vi "14.1 Floss Detection.vi"(8 "ErrI":errorcluster) -> (0 "ErrO":errorcluster)   [LabVIEW 2016]
uses:
  <vilib>/vision/Image Controls.llb/IMAQ Image.ctl
  <vilib>/vision/NI_Vision_Development_Module.lvlib
panel:
  out "Standard  Deviation":sgl format="%#_4g"
  out "Mean Intensity":sgl format="%#_4g"
  in  "Lower Deviation":sgl=64.0
  in  "Upper Deviation":sgl=68.0
  in  "Lower Mean Limitl":sgl=25.0
  in  "Upper Mean Intensity":sgl=28.0
  out "Image":T1(plugin-control)
  in  "Next":bool
  in  "Exit":bool
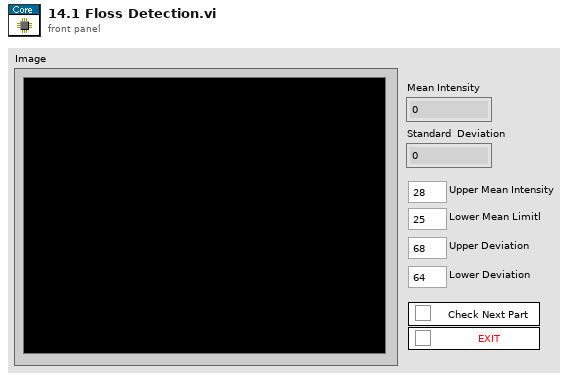
[diagram p1: front panel]
types:
  T1 = typedef "IMAQ Image.ctl" = refnum<image>
  T2 = typedef "IMAQ Rectangle" = cluster{"Left":i32, "Top":i32, "Right":i32, "Bottom":i32, "Rotation":dbl}
  T3 = typedef "IMAQ Coordinate System" = cluster{"Reference System":cluster{"Origin":cluster{"X":sgl, "Y":sgl}, "Angle (deg)":sgl, "Axis Reference":u32}, "Measurement System":cluster{"Origin":cluster{"X":sgl, "Y":sgl}, "Angle (deg)":sgl, "Axis Reference":u32}}
  T4 = cluster{"Tmp":T1, "Src":T1, "Parts":string[], "RefCoord":T3, "MsrCoord":T3, "MsrROI":T2}
  T5 = cluster{"Algorithm":i32, "Minimum Match Score":sgl, "SubPixel Accuracy":bool, "Rotation Angle Ranges":cluster{"Start":sgl, "End":sgl}[], "Show Search Area":bool, "Show Feature Found":bool, "Show Result":bool}
  T6 = cluster{"Mean Intensity":sgl, "Standard  Deviation":sgl, "Minimum Intensity":sgl, "Maximum Intensity":sgl}
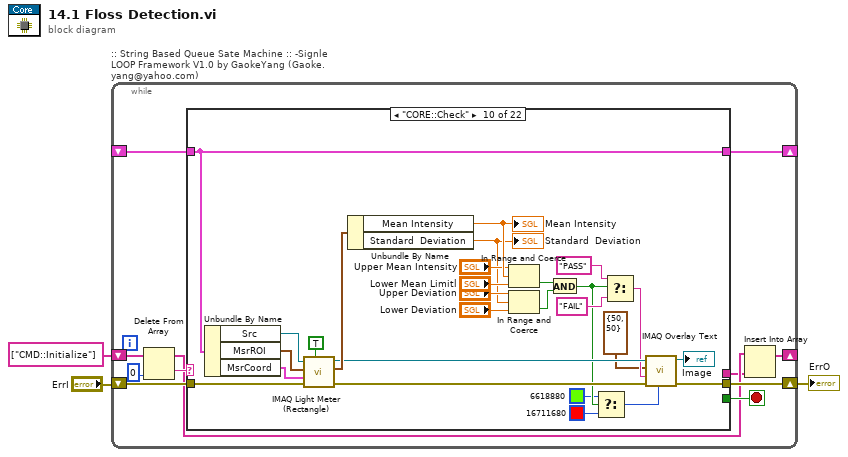
[diagram p0: block diagram]
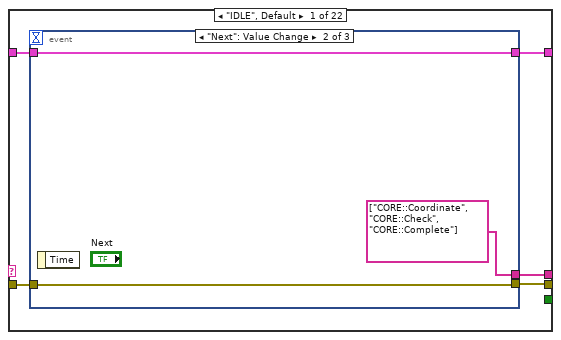
[diagram p2: hidden frame]
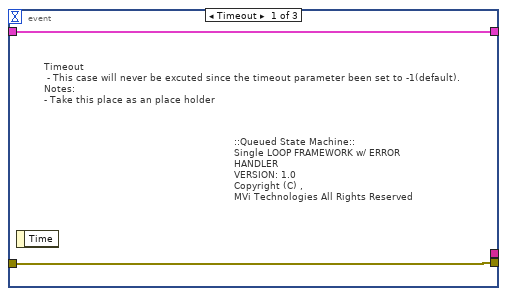
[diagram p3: hidden frame]
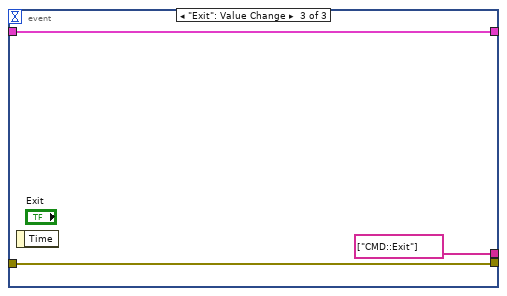
[diagram p4: hidden frame]
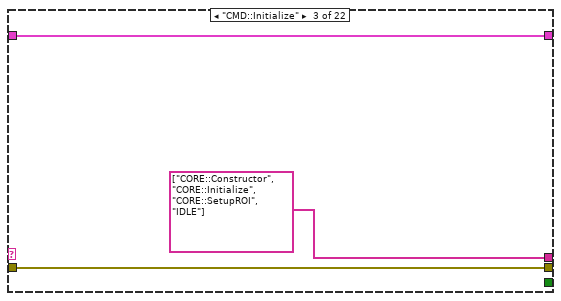
[diagram p6: hidden frame]
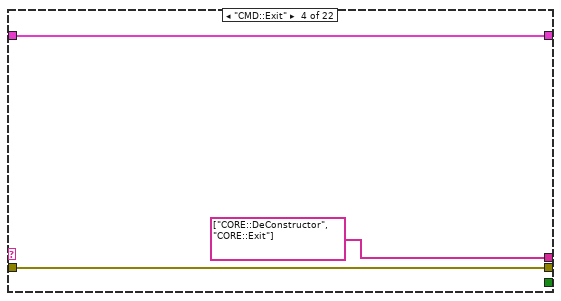
[diagram p7: hidden frame]
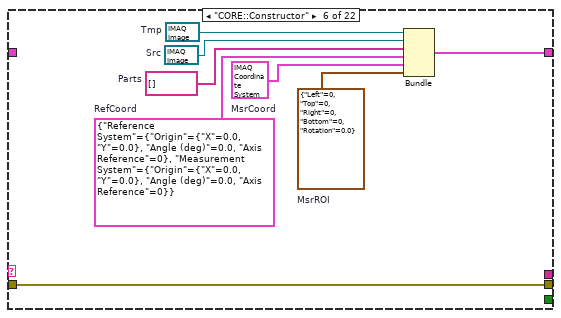
[diagram p9: hidden frame]
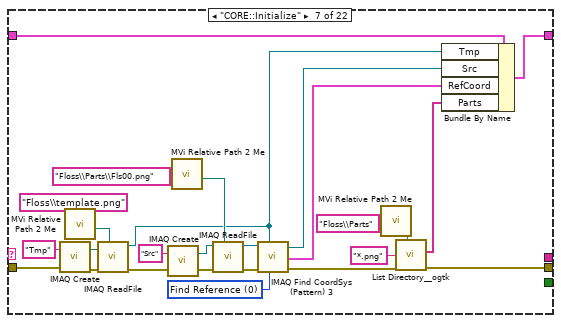
[diagram p10: hidden frame]
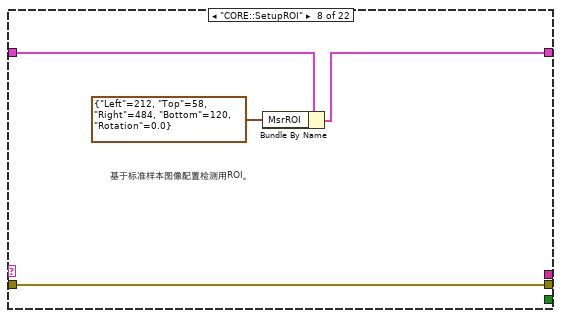
[diagram p11: hidden frame]
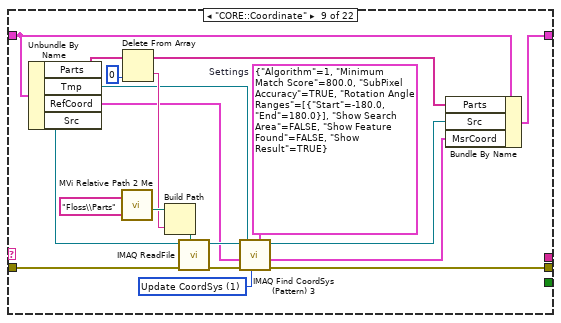
[diagram p12: hidden frame]
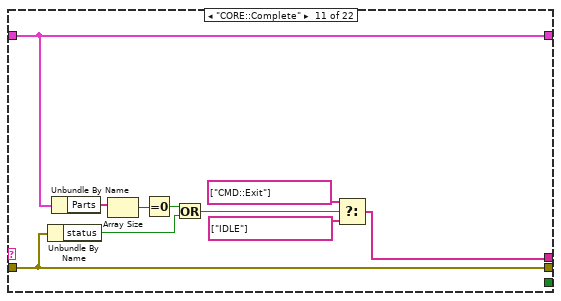
[diagram p13: hidden frame]
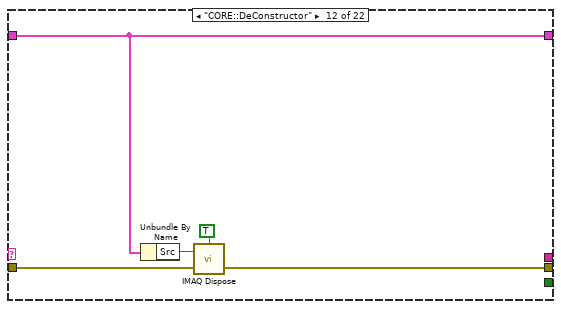
[diagram p14: hidden frame]
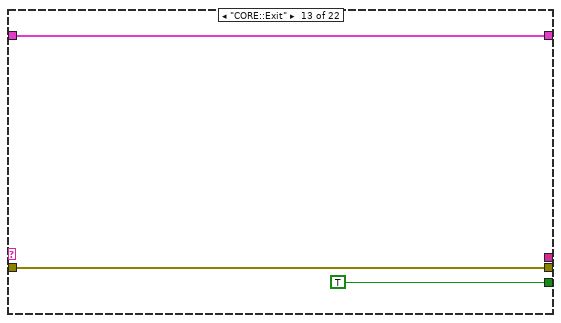
[diagram p15: hidden frame]
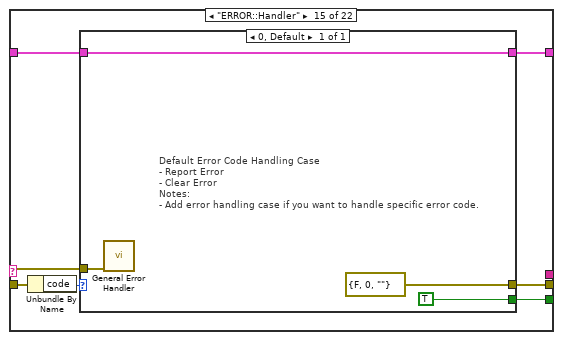
[diagram p17: hidden frame]
diagram:
  n1 = while ":: String Based Queue Sate Machine :: -Signle LOOP Framework V1.0 by GaokeYang (Gaoke.yang@yahoo.com)" {
    shift-right: [w11] -> w3
    shift-left: "ErrI" -> [w9]
    shift-right: [w13] -> _
    shift-left: _ -> [w12]
    shift-right: [w4] -> _
    shift-left: string[] ["CMD::Initialize"] -> [w10]
    stop <- w14 stop-if-true
    n2 = Delete From Array(array=w10, index=0) -> (deleted portion=w8:string, array with subset deleted=w6:string[])  [unwired: 1 in]
    n3 = case shown="\"CORE::Check\"" w8 {
      tunnel: [w18 w29 w31 w34 w37 w44 w61 w72 w83 w114 w128 w136 w138 w142 w145 w153 w155 w157 w160 w162 w164 w165] -> w11
      tunnel: [_ _ _ _ _ _ _ _ _ _ _ _ TRUE _ w144 _ _ _ _ _ _ _] -> w14
      tunnel: w9 -> [w19 w29 w31 w34 w37 w44 w65 w72 w90 w121 w128 w137 w138 w142 w143 w153 w155 w157 w160 w162 w164 w165]
      tunnel: [w16 w28 w32 w35 w36 w45 w68 w75 w87 w122 w129 w135 w139 w141 w146 w154 w156 w158 w159 w161 w163 w166] -> w13
      tunnel: w12 -> [w17 w28 w32 w35 w36 _ w69 w74 w88 w122 w129 w135 w139 w141 w147 w154 w156 w158 w159 w161 w163 w166]
      tunnel: [w15 _ string[] ["CORE::Constructor", "CORE::Initialize", "CORE::SetupROI", "IDLE"] string[] ["CORE::DeConstructor", "CORE::Exit"] _ _ _ _ _ _ w130 _ _ _ _ _ _ _ _ _ _ _] -> w5
      frame "IDLE", Default {
        n4 = event shown="[1] \"Next\": Value Change" {
          selector: _ -> [_ _ _]
          dyn-events: _ -> [_ _ _]
          timeout: _ -> [_ _ _]
          tunnel: [w21 w24 w27] -> w18
          tunnel: w19 -> [w21 w24 w27]
          tunnel: [w20 w23 w26] -> w16
          tunnel: w17 -> [w20 w23 w26]
          tunnel: [_ string[] ["CORE::Coordinate", "CORE::Check", "CORE::Complete"] string[] ["CMD::Exit"]] -> w15
          event Timeout {
            # "Timeout\n - This case will never be excuted since the timeout parameter been set to -1(default).\nNotes:\n- Take this place as an place holder"
            # "::Queued State Machine::\nSingle LOOP FRAMEWORK w/ ERROR HANDLER\nVERSION: 1.0\nCopyright (C) ,\nMVi Technologies All Rights Reserved"
            n5 = event-data() -> ()  [unwired: 1 in, 1 out]
          }
          event "Next": Value Change {
            n6 = event-data() -> ()  [unwired: 1 in, 1 out]
          }
          event "Exit": Value Change {
            n7 = event-data() -> ()  [unwired: 1 in, 1 out]
          }
        }
      }
      frame "-------- Commands ---------" {
      }
      frame "CMD::Initialize" {
      }
      frame "CMD::Exit" {
      }
      frame "------------ Core ------------" {
      }
      frame "CORE::Constructor" {
        w38 = T1 refnum  # Src
        w40 = T2 {"Left"=0, "Top"=0, "Right"=0, "Bottom"=0, "Rotation"=0.0}  # MsrROI
        w41 = T3 {"Reference System"={"Origin"={"X"=0.0, "Y"=0.0}, "Angle (deg)"=0.0, "Axis Reference"=0}, "Measurement System"={"Origin"={"X"=0.0, "Y"=0.0}, "Angle (deg)"=0.0, "Axis Reference"=0}}  # MsrCoord
        w42 = T3 {"Reference System"={"Origin"={"X"=0.0, "Y"=0.0}, "Angle (deg)"=0.0, "Axis Reference"=0}, "Measurement System"={"Origin"={"X"=0.0, "Y"=0.0}, "Angle (deg)"=0.0, "Axis Reference"=0}}  # RefCoord
        w43 = string[] []  # Parts
        w39 = T1 refnum  # Tmp
        n8 = Bundle("Tmp"=w39, "Src"=w38, "Parts"=w43, "RefCoord"=w42, "MsrCoord"=w41, "MsrROI"=w40) -> (w45:T4)  [unwired: 1 in]
      }
      frame "CORE::Initialize" {
        w49 = u16 0 items=["Find Reference", "Update CoordSys"] ("Mode")
        n9 = call "IMAQ Create"("Image Name"="Tmp", "error in (no error)"=w65) -> ("Src"=w67:T1, "error out"=w66:errorcluster)  [unwired: 3 in]
        n10 = call "MVi Relative Path 2 Me.vi"("Relative Path"="Floss\\template.png" ("name or relative path")) -> ("Appended Dir"=w52:path)  [unwired: 5 in, 1 out]
        n11 = call "IMAQ ReadFile"("File Path"=w52, "error in (no error)"=w66, "Image"=w67) -> ("error out"=w57:errorcluster, "Image Out"=w48:T1)  [unwired: 4 in, 3 out]
        n12 = call "IMAQ Create"("Image Name"="Src", "error in (no error)"=w57) -> ("Src"=w54:T1, "error out"=w55:errorcluster)  [unwired: 3 in]
        n13 = call "MVi Relative Path 2 Me.vi"("Relative Path"="Floss\\Parts\\Fls00.png" ("name or relative path")) -> ("Appended Dir"=w51:path)  [unwired: 5 in, 1 out]
        n14 = call "IMAQ ReadFile"("File Path"=w51, "error in (no error)"=w55, "Image"=w54) -> ("error out"=w56:errorcluster, "Image Out"=w50:T1)  [unwired: 4 in, 3 out]
        n15 = call "IMAQ Find CoordSys (Pattern) 3"("Mode"=w49, "Template"=w48, "error in"=w56, "Image"=w50) -> ("error out"=w46:errorcluster, "Coordinate System Out"=w59:T3, "Image Out"=w47:T1)  [unwired: 3 in, 2 out]
        n16 = call "MVi Relative Path 2 Me.vi"("Relative Path"="Floss\\Parts" ("name or relative path")) -> ("Appended Dir"=w63:path)  [unwired: 5 in, 1 out]
        n17 = call "List Directory__ogtk.vi"("error in (no error)"=w46, "pattern"="*.png", "directory path"=w63) -> ("error out"=w61:errorcluster, "file names"=w60:string[])  [unwired: 1 in, 2 out]
        n18 = Bundle By Name(cluster=w69, "Tmp"=w48, "Src"=w47, "RefCoord"=w59, "Parts"=w60) -> (w68:T4)
      }
      frame "CORE::SetupROI" {
        # "基于标准样本图像配置检测用ROI。"
        n19 = Bundle By Name(cluster=w74, "MsrROI"=T2 {"Left"=212, "Top"=58, "Right"=484, "Bottom"=120, "Rotation"=0.0} ("Rectangle")) -> (w75:T4)
      }
      frame "CORE::Coordinate" {
        w80 = T5 {"Algorithm"=1, "Minimum Match Score"=800.0, "SubPixel Accuracy"=TRUE, "Rotation Angle Ranges"=[{"Start"=-180.0, "End"=180.0}], "Show Search Area"=FALSE, "Show Feature Found"=FALSE, "Show Result"=TRUE}  # Settings
        w84 = u16 1 items=["Find Reference", "Update CoordSys"] ("Mode")
        n20 = Unbundle By Name(w88) -> ("Parts"=w76:string[], "Tmp"=w77:T1, "RefCoord"=w78:T3, "Src"=w81:T1)
        n21 = call "MVi Relative Path 2 Me.vi"("Relative Path"="Floss\\Parts" ("name or relative path")) -> ("Appended Dir"=w94:path)  [unwired: 5 in, 1 out]
        n22 = Delete From Array(array=w76, index=0) -> (deleted portion=w92:string, array with subset deleted=w89:string[])  [unwired: 1 in]
        n23 = Build Path(base path=w94, name or relative path=w92) -> (appended path=w91:path)
        n24 = call "IMAQ ReadFile"("File Path"=w91, "error in (no error)"=w90, "Image"=w81) -> ("error out"=w85:errorcluster, "Image Out"=w86:T1)  [unwired: 4 in, 3 out]
        n25 = call "IMAQ Find CoordSys (Pattern) 3"("Settings"=w80, "Mode"=w84, "Template"=w77, "error in"=w85, "Coordinate System In"=w78, "Image"=w86) -> ("error out"=w83:errorcluster, "Coordinate System Out"=w82:T3, "Image Out"=w79:T1)  [unwired: 1 in, 2 out]
        n26 = Bundle By Name(cluster=w88, "Parts"=w89, "Src"=w79, "MsrCoord"=w82) -> (w87:T4)
      }
      frame "CORE::Check" {
        n27 = Unbundle By Name(w122) -> ("Src"=w118:T1, "MsrROI"=w119:T2, "MsrCoord"=w120:T3)
        n28 = call "IMAQ Light Meter (Rectangle)"("Show Search Area"=TRUE, "error in (no error)"=w121, "Coordinate System"=w120, "Rectangle"=w119, "Image"=w118) -> ("error out"=w115:errorcluster, "Gray Level Intensities"=w116:T6, "Image Out"=w113:T1)  [unwired: 2 in, 2 out]
        n29 = Unbundle By Name(w116) -> ("Mean Intensity"=w112:sgl, "Standard  Deviation"=w107:sgl)
        "Mean Intensity" <- w112
        "Standard  Deviation" <- w107
        n30 = In Range and Coerce(upper limit="Upper Mean Intensity", x=w112, lower limit="Lower Mean Limitl") -> (In Range?=w106:bool)  [unwired: 1 out]
        n31 = In Range and Coerce(upper limit="Upper Deviation", x=w107, lower limit="Lower Deviation") -> (In Range?=w105:bool)  [unwired: 1 out]
        n32 = And(x=w106, y=w105) -> (x .and. y?=w101:bool)
        n33 = Select(t=u32 6618880 ("Text Color (black)"), s=w101, f=u32 16711680 ("Text Color (black)")) -> (s? t:f=w98:u32)
        n34 = Select(t="PASS", s=w101, f="FAIL") -> (s? t:f=w102:string)
        n35 = call "IMAQ Overlay Text"("Text Color (black)"=w98, "error in (no error)"=w115, "String"=w102, "Origin"=cluster{"X":i32, "Y":i32} {"X"=50, "Y"=50}, "Image"=w113) -> ("error out"=w114:errorcluster, "Image Out"=→"Image":T1)  [unwired: 5 in]
      }
      frame "CORE::Complete" {
        n36 = Unbundle By Name(w128) -> ("status"=w124:bool)
        n37 = Unbundle By Name(w129) -> ("Parts"=w127:string[])
        n38 = Array Size(array=w127) -> (size(s)=w126:i32)
        n39 = Equal To 0?(x=w126) -> (x = 0?=w125:bool)
        n40 = Or(x=w125, y=w124) -> (x .or. y?=w123:bool)
        n41 = Select(t=string[] ["CMD::Exit"], s=w123, f=string[] ["IDLE"]) -> (s? t:f=w130:string[])
      }
      frame "CORE::DeConstructor" {
        n42 = Unbundle By Name(w135) -> ("Src"=w134:T1)
        n43 = call "IMAQ Dispose"("All Images? (No)"=TRUE, "Image"=w134, "error in (no error)"=w137) -> ("error out"=w136:errorcluster)  [unwired: 3 in]
      }
      frame "CORE::Exit" {
      }
      frame "-------- Error Handle--------" {
      }
      frame "ERROR::Handler" {
        n44 = Unbundle By Name(w143) -> ("code"=w148:i32)
        n45 = case shown="0, Default" w148 {
          tunnel: [w152] -> w146
          tunnel: w147 -> [w152]
          tunnel: [errorcluster {"status"=FALSE, "code"=0, "source"=""} ("error out")] -> w145
          tunnel: [TRUE] -> w144
          tunnel: w143 -> [w150]
          frame 0, Default {
            # "Default Error Code Handling Case\n- Report Error\n- Clear Error \nNotes:\n- Add error handling case if you want to handle specific error code."
            n46 = call <vilib>:"General Error Handler.vi"("error in (no error)"=w150) -> ()  [unwired: 10 in, 5 out]
          }
        }
      }
      frame "------------  GUI  ------------" {
      }
      frame "GUI::Initialize" {
      }
      frame "GUI::SetCusor" {
      }
      frame "GUI::SetMenu" {
      }
      frame "------------ USER -----------" {
      }
      frame "USER::Case1" {
      }
      frame "USER::Case2" {
      }
    }
    n47 = Insert Into Array(array=w6, new element=w5) -> (w4:string[])  [unwired: 1 in]
  }
  "ErrO" <- w3
